vi "Listener VI.vi"(5 "AK?":bool, 7 "Operation":T1, 8 "error in (no error)":errorcluster, 11 "Listener.lvclass":refnum<class "Listener.lvclass">) -> (0 "error out":errorcluster, 3 "Listener Out.lvclass":refnum<class "Listener.lvclass">)   [LabVIEW 2019]
doc: "Reads/Writes data using the specified protocol.\nInput: \nListener Object\nMessage: The \"packet\" which will be sent through the selected protocol\nOpeartion: Read/Write operation on the specified protocol\nAK?: Special parameter for AK TCP and RS-xxx protocol"
uses:
  Listener.lvclass
  ListenerClassControls/Operation Ctl.ctl
panel:
  in  "Message":string
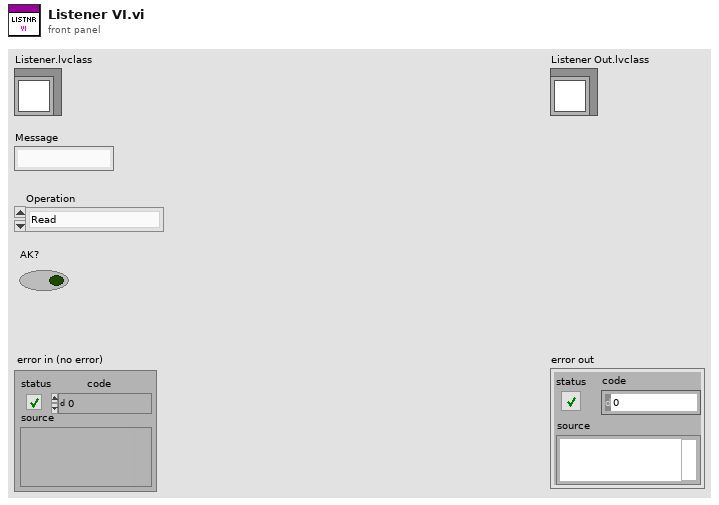
[diagram p1: front panel]
types:
  T1 = typedef "Operation Ctl.ctl" = enum16{"Read", "Write"}
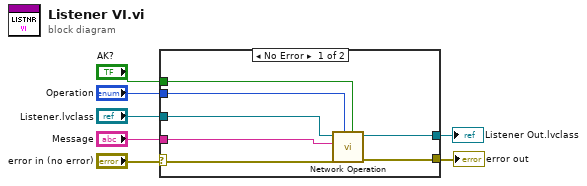
[diagram p0: block diagram]
diagram:
  n1 = case shown="No Error" "error in (no error)" {
    selector: "error in (no error)" -> [w11 w15]
    tunnel: "Listener.lvclass" -> [w14 w16]
    tunnel: [w13 w15] -> w7
    tunnel: [w12 w16] -> w6
    tunnel: "Operation" -> [w10 _]
    tunnel: "AK?" -> [w9 _]
    tunnel: "Message" -> [w8 _]
    frame No Error {
      n2 = call "Network Operation.vi"("AK?"=w9, "Operation"=w10, "error in (no error)"=w11, "Message"=w8, "Listener In.lvclass"=w14) -> ("error out"=w13:errorcluster, "Listener Out.lvclass"=w12:refnum<class "Listener.lvclass">)  [unwired: 5 in]
    }
    frame Error {
    }
  }
  "error out" <- w7
  "Listener Out.lvclass" <- w6
